vi "remote reg store.vi"(4 "catch? in":bool, 6 "dir in":i32, 7 "height in":dbl, 8 "reg":i32, 9 "dt":dbl, 10 "delay timer in":i32, 11 "PC in":i32) -> (0 "delay timer out":i32, 1 "PC out":i32, 2 "height out":dbl, 3 "dir out":i32, 5 "catch? out":bool)   [LabVIEW 2019]
uses:
  ctl/height.ctl
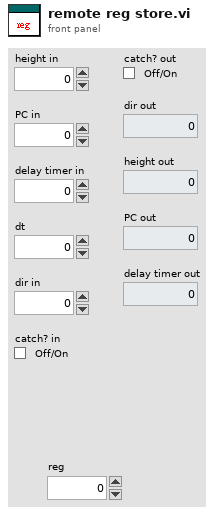
[diagram p1: front panel]
types:
  T1 = typedef "height.ctl" = enum16{"IDLE", "recycle pre-catch", "recycle catch", "recycle zone", "vision height", "box 1", "box 2", "box 3", "box 1 pre", "box 2 pre", "box 3 pre", "reg 1", "reg 2", "reg 1 pre", "reg 2 pre", "put 1", "put 2", "put 3"}
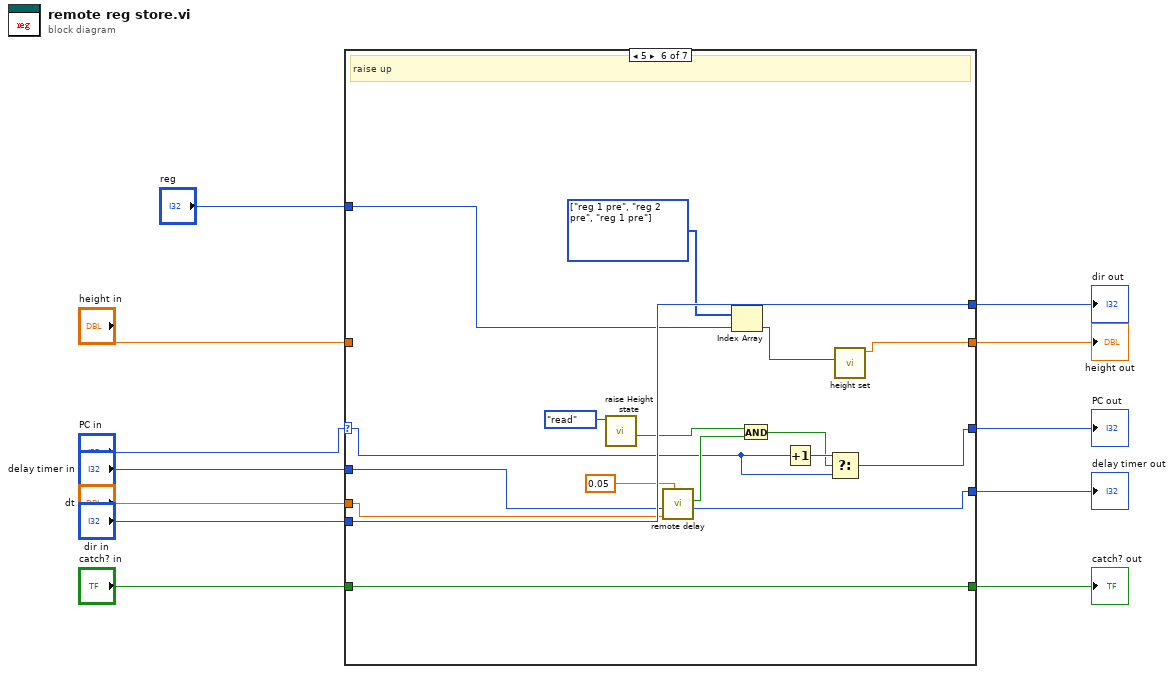
[diagram p0: block diagram]
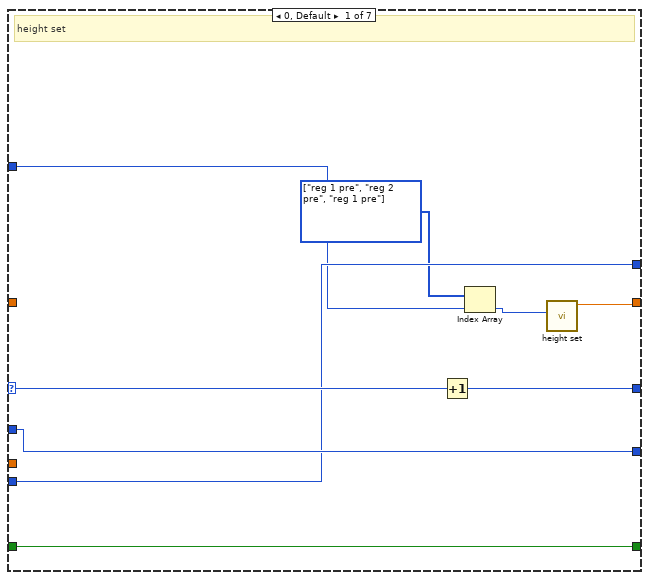
[diagram p2: hidden frame]
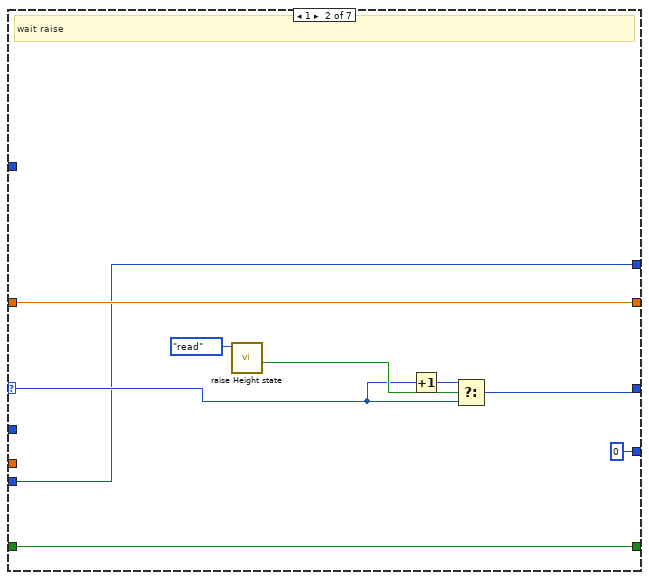
[diagram p3: hidden frame]
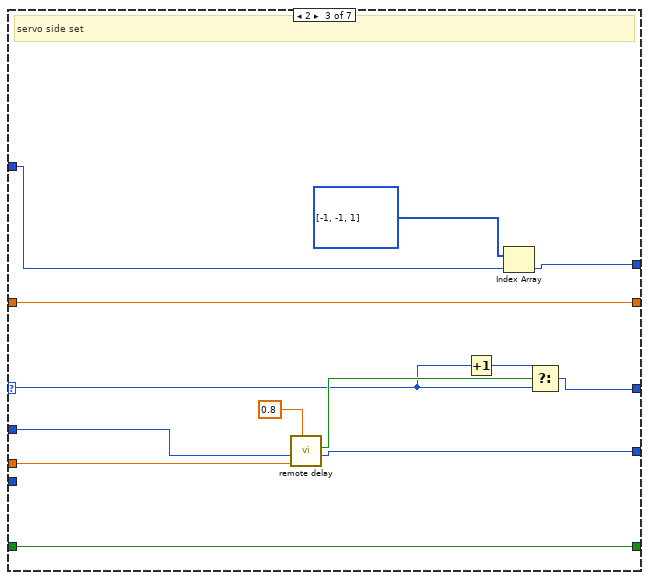
[diagram p4: hidden frame]
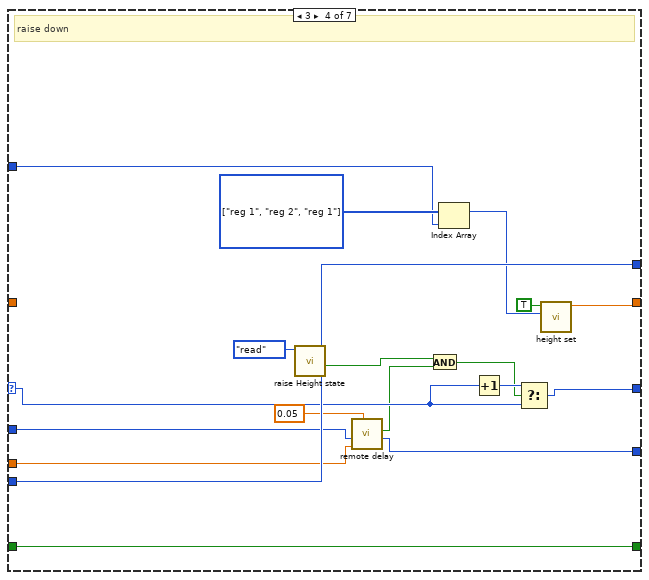
[diagram p5: hidden frame]
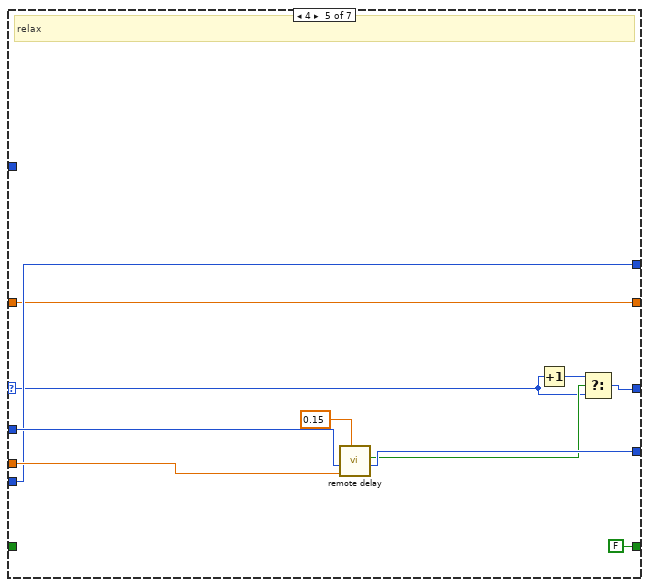
[diagram p6: hidden frame]
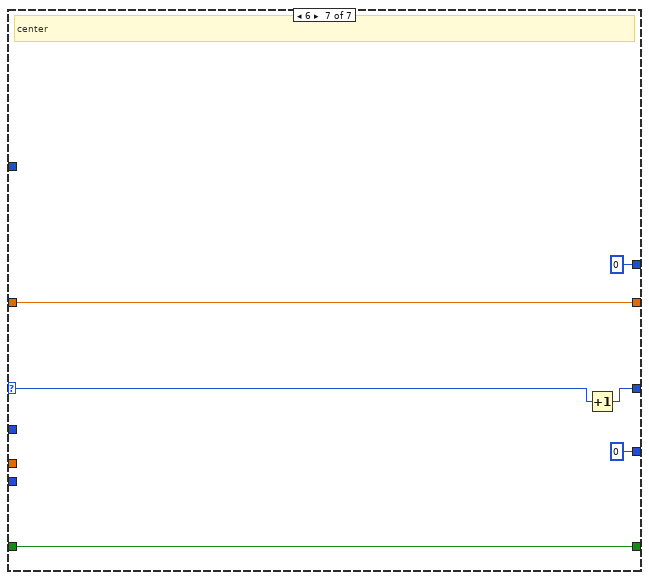
[diagram p7: hidden frame]
diagram:
  n1 = case shown="5" "PC in" {
    selector: "PC in" -> [w19 w25 w36 w54 w62 w81 w94]
    tunnel: "delay timer in" -> [w20 _ w42 w51 w70 w78 _]
    tunnel: [w21 w30 w43 w61 w67 w89 w91] -> w4
    tunnel: "height in" -> [_ w30 w43 _ w67 _ w91]
    tunnel: [w20 0 ("Delay counter") w41 w52 w71 w79 0 ("i out")] -> w6
    tunnel: [w18 w27 w35 w53 w64 w80 w95] -> w12
    tunnel: [w16 w23 w33 w58 w68 w88 0] -> w7
    tunnel: "dt" -> [_ _ w40 w50 w69 w77 _]
    tunnel: "dir in" -> [w16 w23 _ w58 w68 w88 _]
    tunnel: "catch? in" -> [w17 w22 w34 w57 _ w76 w92]
    tunnel: [w17 w22 w34 w57 FALSE w76 w92] -> w11
    tunnel: "reg" -> [w14 _ w31 w44 _ w73 _]
    frame 0, Default {
      w15 = T1[] [enum."reg 1 pre", enum."reg 2 pre", enum."reg 1 pre"] items=["IDLE", "recycle pre-catch", "recycle catch", "recycle zone", "vision height", "box 1", "box 2", "box 3", "box 1 pre", "box 2 pre", "box 3 pre", "reg 1", "reg 2", "reg 1 pre", "reg 2 pre", "put 1", "put 2", "put 3"] ("height name")
      # "height set"
      n2 = Increment(x=w19) -> (x+1=w18:i32)
      n3 = Index Array(array=w15, index=w14) -> (element=w13:T1)
      n4 = call "height set.vi"("height name"=w13) -> ("Numeric"=w21:dbl)  [unwired: 10 in]
    }
    frame 1 {
      # "wait raise"
      n5 = call "raise Height state.vi"("Enum"=enum16{"read", "write"}."read") -> ("read"=w28:bool)  [unwired: 9 in, 1 out]
      n6 = Increment(x=w25) -> (x+1=w26:i32)
      n7 = Select(t=w26, s=w28, f=w25) -> (s? t:f=w27:i32)
    }
    frame 2 {
      # "servo side set"
      n8 = call "remote delay.vi"("second"=0.8, "dt(s)"=w40, "i"=w42) -> ("i out"=w41:i32, "finish?"=w38:bool)  [unwired: 7 in]
      n9 = Increment(x=w36) -> (x+1=w37:i32)
      n10 = Index Array(array=i32[] [-1, -1, 1], index=w31) -> (element=w33:i32)
      n11 = Select(t=w37, s=w38, f=w36) -> (s? t:f=w35:i32)
    }
    frame 3 {
      w60 = T1[] [enum."reg 1", enum."reg 2", enum."reg 1"] items=["IDLE", "recycle pre-catch", "recycle catch", "recycle zone", "vision height", "box 1", "box 2", "box 3", "box 1 pre", "box 2 pre", "box 3 pre", "reg 1", "reg 2", "reg 1 pre", "reg 2 pre", "put 1", "put 2", "put 3"] ("height name")
      # "raise down"
      n12 = call "raise Height state.vi"("Enum"=enum16{"read", "write"}."read") -> ("read"=w48:bool)  [unwired: 9 in, 1 out]
      n13 = call "remote delay.vi"("second"=0.05, "dt(s)"=w50, "i"=w51) -> ("i out"=w52:i32, "finish?"=w47:bool)  [unwired: 7 in]
      n14 = And(x=w48, y=w47) -> (x .and. y?=w46:bool)
      n15 = Index Array(array=w60, index=w44) -> (element=w45:T1)
      n16 = Increment(x=w54) -> (x+1=w55:i32)
      n17 = Select(t=w55, s=w46, f=w54) -> (s? t:f=w53:i32)
      n18 = call "height set.vi"("height name"=w45, "plus in"=TRUE) -> ("Numeric"=w61:dbl)  [unwired: 9 in]
    }
    frame 4 {
      # "relax"
      n19 = call "remote delay.vi"("second"=0.15, "dt(s)"=w69, "i"=w70) -> ("i out"=w71:i32, "finish?"=w65:bool)  [unwired: 7 in]
      n20 = Increment(x=w62) -> (x+1=w63:i32)
      n21 = Select(t=w63, s=w65, f=w62) -> (s? t:f=w64:i32)
    }
    frame 5 {
      w75 = T1[] [enum."reg 1 pre", enum."reg 2 pre", enum."reg 1 pre"] items=["IDLE", "recycle pre-catch", "recycle catch", "recycle zone", "vision height", "box 1", "box 2", "box 3", "box 1 pre", "box 2 pre", "box 3 pre", "reg 1", "reg 2", "reg 1 pre", "reg 2 pre", "put 1", "put 2", "put 3"] ("height name")
      # "raise up"
      n22 = call "raise Height state.vi"("Enum"=enum16{"read", "write"}."read") -> ("read"=w84:bool)  [unwired: 9 in, 1 out]
      n23 = call "remote delay.vi"("second"=0.05, "dt(s)"=w77, "i"=w78) -> ("i out"=w79:i32, "finish?"=w83:bool)  [unwired: 7 in]
      n24 = Index Array(array=w75, index=w73) -> (element=w74:T1)
      n25 = And(x=w84, y=w83) -> (x .and. y?=w82:bool)
      n26 = Increment(x=w81) -> (x+1=w86:i32)
      n27 = Select(t=w86, s=w82, f=w81) -> (s? t:f=w80:i32)
      n28 = call "height set.vi"("height name"=w74) -> ("Numeric"=w89:dbl)  [unwired: 10 in]
    }
    frame 6 {
      # "center"
      n29 = Increment(x=w94) -> (x+1=w95:i32)
    }
  }
  "PC out" <- w12
  "catch? out" <- w11
  "dir out" <- w7
  "delay timer out" <- w6
  "height out" <- w4
